vi "MTS_ToColorImage.vi"(0 "Data In":u32[](array[numeric]), 1 "Reset":bool, 2 "Image Array In":i32[][][](array[numeric]), 5 "Data Count":i32, 7 "TCSPC Binning":i32[][](array[numeric]), 9 "Pixel Time (Laser Pulses)":i32, 11 "Trace Bins":i32=25) -> (3 "Image Array Out":i32[][][](array[numeric]), 6 "Total Photon Count":u64[](array[numeric]), 8 "Trigger Times":u64[](array[numeric]), 13 "Total Oveflow Count":u64, 14 "Num Records Total":i32, 15 "Traces":i32[][](array[numeric]))   [LabVIEW 8.6]
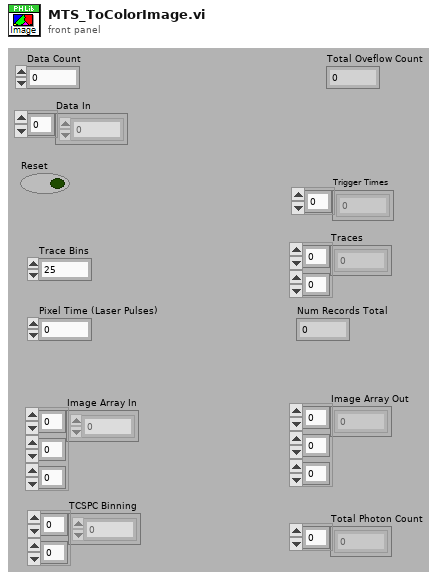
[diagram p1: front panel]
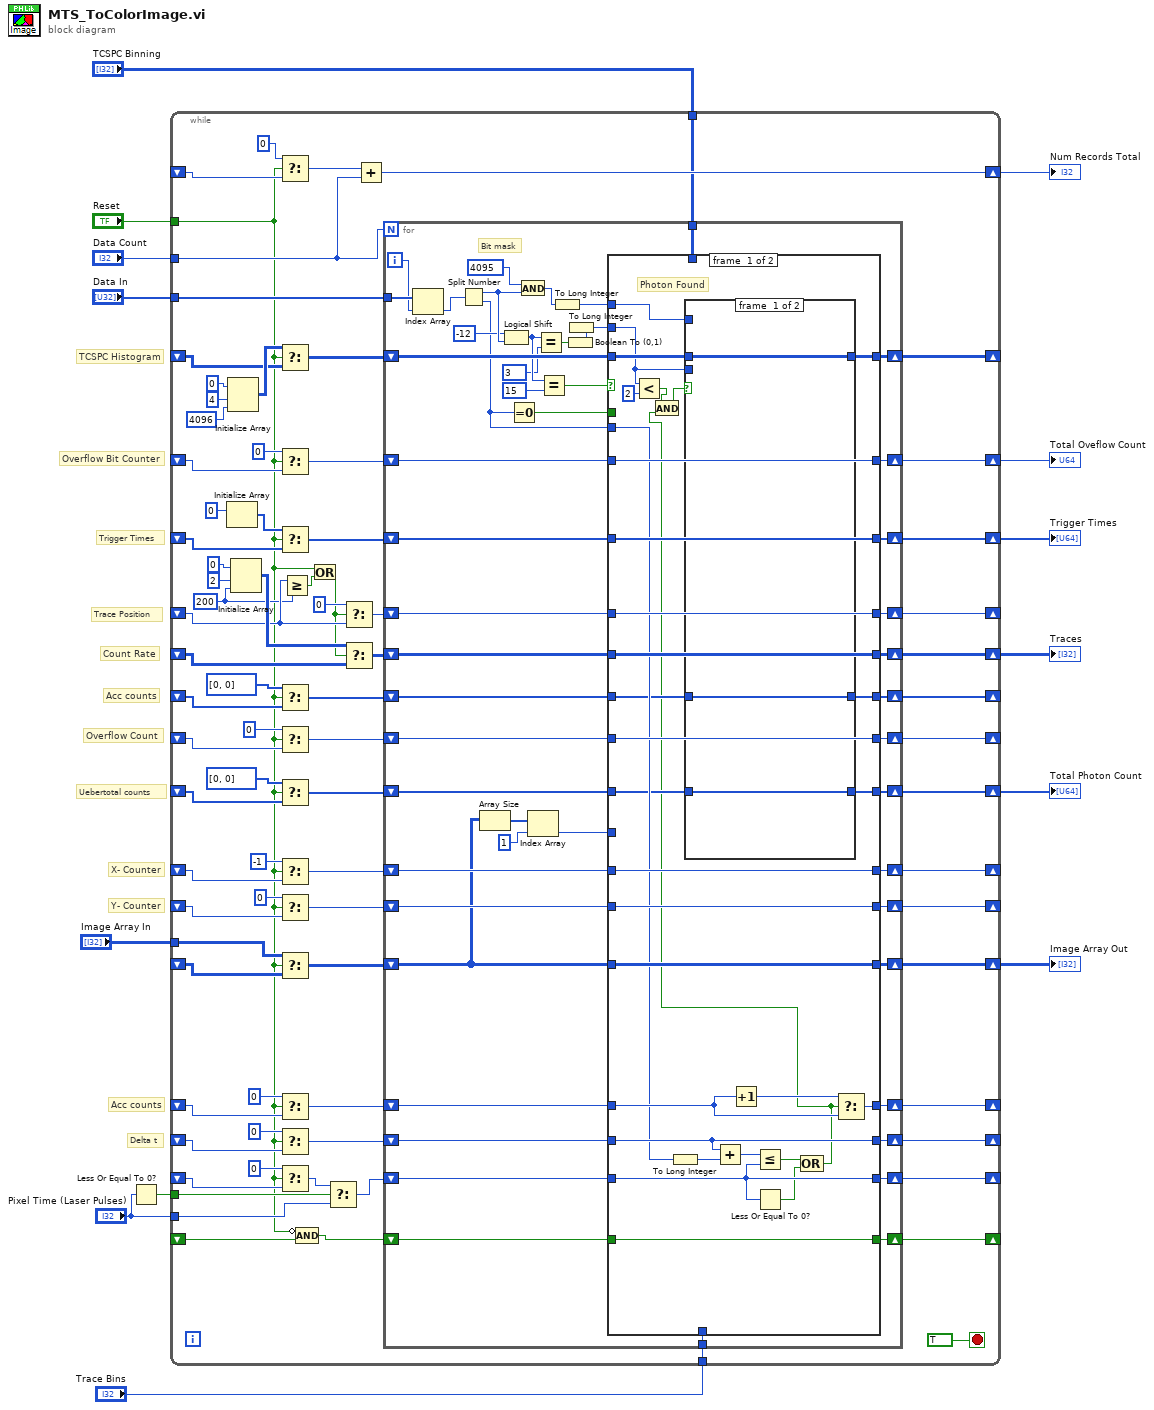
[diagram p0: block diagram]
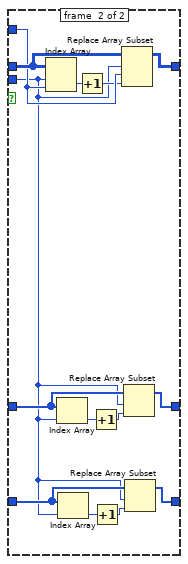
[diagram p2: hidden frame]
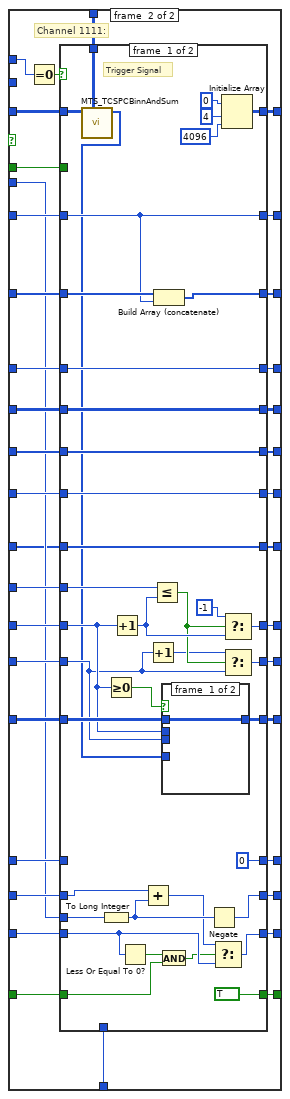
[diagram p3: hidden frame]
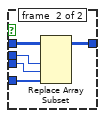
[diagram p4: hidden frame]
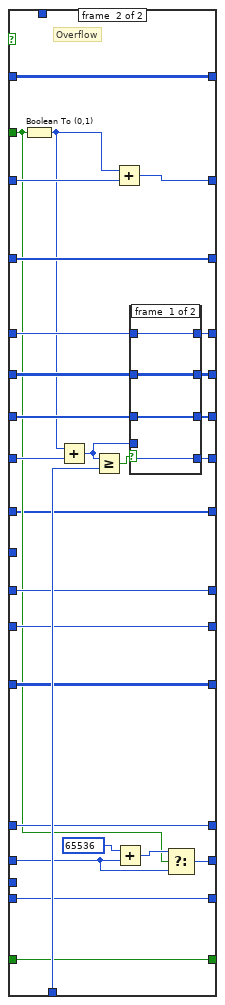
[diagram p5: hidden frame]
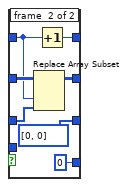
[diagram p6: hidden frame]
diagram:
  # "Uebertotal counts"
  # "Y- Counter"
  # "X- Counter"
  # "Delta t"
  # "Acc counts"
  # "Trace Position"
  # "Overflow Count"
  # "Acc counts"
  # "Count Rate"
  # "Trigger Times"
  # "TCSPC Histogram"
  # "Overflow Bit Counter"
  n1 = Less Or Equal To 0?(x="Pixel Time (Laser Pulses)") -> (x <= 0?=w3:bool)
  n2 = while {
    tunnel: "Data In" -> [w93]
    shift-right: [w94] -> _
    shift-left: _ -> [w89]
    tunnel: "Reset" -> [w16]
    shift-right: [w86] -> w5
    shift-left: _ -> [w85]
    shift-right: [w81] -> w12
    shift-left: _ -> [w80]
    shift-right: [w76] -> w10
    shift-left: _ -> [w75]
    shift-right: [w73] -> _
    shift-left: _ -> [w72]
    shift-right: [w70] -> _
    shift-left: _ -> [w69]
    tunnel: "Trace Bins" -> [w68]
    shift-right: [w65] -> _
    shift-left: _ -> [w63]
    shift-right: [w59] -> w8
    shift-left: _ -> [w58]
    tunnel: "Image Array In" -> [w61]
    shift-right: [w54] -> _
    shift-left: _ -> [w52]
    shift-right: [w53] -> _
    shift-left: _ -> [w51]
    shift-right: [w46] -> _
    shift-left: _ -> [w44]
    shift-right: [w45] -> _
    shift-left: _ -> [w43]
    tunnel: "Data Count" -> [w38]
    shift-right: [w37] -> w6
    shift-left: _ -> [w40]
    shift-right: [w28] -> w4
    shift-left: _ -> [w27]
    shift-right: [w23] -> _
    shift-left: _ -> [w20]
    tunnel: w3 -> [w25]
    tunnel: "Pixel Time (Laser Pulses)" -> [w24]
    shift-right: [w19] -> _
    shift-left: _ -> [w18]
    tunnel: "TCSPC Binning" -> [w15]
    stop <- TRUE stop-if-true
    w34 = 200 ("dimension size")
    n3 = Initialize Array(u64 0 ("element")) -> (w83:u64[])  [unwired: 1 out]
    n4 = Initialize Array(0 ("element"), 4 ("dimension size"), 4096 ("dimension size")) -> (w90:i32[][])
    n5 = Initialize Array(0 ("element"), 2 ("dimension size"), w34) -> (w78:i32[][])
    n6 = Select(t=0 ("Data Count 2"), s=w16, f=w40) -> (s? t:f=w39:i32)
    n7 = Select(t=w90, s=w16, f=w89) -> (s? t:f=w91:i32[][])
    n8 = Select(t=u64 0, s=w16, f=w85) -> (s? t:f=w87:u64)
    n9 = Select(t=w83, s=w16, f=w80) -> (s? t:f=w82:u64[])
    n10 = Select(t=u32[] [0, 0] ("initialized array"), s=w16, f=w72) -> (s? t:f=w74:u32[])
    n11 = Select(t=u32 0, s=w16, f=w69) -> (s? t:f=w71:u32)
    n12 = Select(t=u64[] [0, 0] ("initialized array"), s=w16, f=w27) -> (s? t:f=w29:u64[])
    n13 = Select(t=-1, s=w16, f=w44) -> (s? t:f=w48:i32)
    n14 = Select(t=0, s=w16, f=w43) -> (s? t:f=w47:i32)
    n15 = Select(t=w61, s=w16, f=w58) -> (s? t:f=w60:i32[][][])
    n16 = Select(t=0, s=w16, f=w52) -> (s? t:f=w56:i32)
    n17 = Select(t=0, s=w16, f=w51) -> (s? t:f=w55:i32)
    n18 = Select(t=0, s=w16, f=w20) -> (s? t:f=w22:i32)
    n19 = Greater Or Equal?(x=w63, y=w34) -> (x >= y?=w64:bool)
    n20 = Compound Arithmetic op=AND(invert w16, w18) -> (w17:bool)
    n21 = Or(x=w16, y=w64) -> (x .or. y?=w62:bool)
    n22 = Select(t=w22, s=w25, f=w24) -> (s? t:f=w26:i32)
    n23 = Select(t=0, s=w62, f=w63) -> (s? t:f=w66:i32)
    n24 = Select(t=w78, s=w62, f=w75) -> (s? t:f=w77:i32[][])
    n25 = Add(x=w39, y=w38) -> (x+y=w37:i32)
    n26 = for {
      N: w38 -> [_]
      tunnel: w93 -> [w110]
      shift-right: [w143] -> w94
      shift-left: w91 -> [w145]
      shift-right: [w137] -> w86
      shift-left: w87 -> [w138]
      shift-right: [w135] -> w81
      shift-left: w82 -> [w136]
      shift-right: [w130] -> w76
      shift-left: w77 -> [w131]
      shift-right: [w132] -> w73
      shift-left: w74 -> [w133]
      shift-right: [w128] -> w70
      shift-left: w71 -> [w129]
      tunnel: w68 -> [w127]
      shift-right: [w125] -> w65
      shift-left: w66 -> [w126]
      shift-right: [w124] -> w59
      shift-left: w60 -> [w116]
      shift-right: [w122] -> w54
      shift-left: w56 -> [w123]
      shift-right: [w120] -> w53
      shift-left: w55 -> [w121]
      shift-right: [w117] -> w46
      shift-left: w48 -> [w118]
      shift-right: [w113] -> w45
      shift-left: w47 -> [w119]
      shift-right: [w101] -> w28
      shift-left: w29 -> [w102]
      shift-right: [w100] -> w23
      shift-left: w26 -> [w112]
      shift-right: [w99] -> w19
      shift-left: w17 -> [w98]
      tunnel: w15 -> [w96]
      i -> [w109]
      # "Bit mask"
      n27 = Index Array(array=w110, index=w109) -> (element=w108:u32)
      n28 = Split Number(x=w108) -> (hi(x)=w142:u16, lo(x)=w111:u16)
      n29 = Array Size(array=w116) -> (size(s)=w115:i32[])
      n30 = Logical Shift(y=i8 -12, x=w142) -> (x << y=w107:u16)
      n31 = Equal To 0?(x=w111) -> (x = 0?=w134:bool)
      n32 = And(x=u16 4095, y=w142) -> (x .and. y?=w146:u16)
      n33 = Index Array(array=w115, index=1) -> (element=w114:i32)
      n34 = Equal?(x=w107, y=u16 3) -> (x = y?=w105:bool)
      n35 = Equal?(x=w107, y=u16 15) -> (x = y?=w139:bool)
      n36 = To Long Integer(number=w146) -> (32bit integer=w144:i32)
      n37 = Boolean To (0,1)(Boolean=w105) -> (0, 1=w104:i16)
      n38 = To Long Integer(number=w104) -> (32bit integer=w103:i32)
      n39 = case shown="True" w139 {
        tunnel: w145 -> [w178 w198]
        tunnel: w144 -> [w161 w211]
        tunnel: [w177 w197] -> w143
        tunnel: w103 -> [w158 _]
        tunnel: w138 -> [w176 w231]
        tunnel: [w176 w230] -> w137
        tunnel: w136 -> [w175 w229]
        tunnel: [w175 w228] -> w135
        tunnel: w134 -> [_ w227]
        tunnel: w133 -> [w160 w225]
        tunnel: [w159 w221] -> w132
        tunnel: w131 -> [w174 w224]
        tunnel: [w174 w220] -> w130
        tunnel: w129 -> [w173 w226]
        tunnel: [w173 w222] -> w128
        tunnel: w127 -> [_ w223]
        tunnel: w126 -> [w172 w219]
        tunnel: [w172 w218] -> w125
        tunnel: w116 -> [w171 w216]
        tunnel: [w171 w217] -> w124
        tunnel: w123 -> [w170 w212]
        tunnel: [w169 w213] -> w122
        tunnel: w121 -> [w168 w215]
        tunnel: [w168 w214] -> w120
        tunnel: w119 -> [w167 w210]
        tunnel: w118 -> [w166 w209]
        tunnel: [w166 w208] -> w117
        tunnel: w114 -> [_ w207]
        tunnel: [w167 w206] -> w113
        tunnel: w112 -> [w154 w202]
        tunnel: w111 -> [w163 w205]
        tunnel: w102 -> [w156 w204]
        tunnel: [w155 w203] -> w101
        tunnel: [w154 w201] -> w100
        tunnel: [w151 w200] -> w99
        tunnel: w98 -> [w151 w199]
        tunnel: w96 -> [_ w196]
        frame #0 {
          # "Photon Found"
          n40 = Less?(x=w158, y=2) -> (x < y?=w150:bool)
          n41 = To Long Integer(number=w163) -> (32bit integer=w162:i32)
          n42 = Add(x=w168, y=w162) -> (x+y=w164:i32)
          n43 = Increment(x=w170) -> (x+1=w165:i32)
          n44 = Less Or Equal?(x=w164, y=w154) -> (x <= y?=w153:bool)
          n45 = Less Or Equal To 0?(x=w154) -> (x <= 0?=w152:bool)
          n46 = Compound Arithmetic op=OR(w153, w152) -> (w148:bool)
          n47 = And(x=w150, y=w148) -> (x .and. y?=w149:bool)
          n48 = case shown="True" w149 {
            tunnel: w178 -> [w181 w195]
            tunnel: [w181 w194] -> w177
            tunnel: w161 -> [_ w193]
            tunnel: w158 -> [_ w182]
            tunnel: w160 -> [w180 w192]
            tunnel: [w180 w191] -> w159
            tunnel: w156 -> [w179 w184]
            tunnel: [w179 w183] -> w155
            frame #0 {
            }
            frame #1 {
              n49 = Index Array(array=w195, index (row)=w182, index (col)=w193) -> (element=w190:i32)
              n50 = Index Array(array=w192, index=w182) -> (element=w188:u32)
              n51 = Index Array(array=w184, index=w182) -> (element=w186:u64)
              n52 = Increment(x=w190) -> (x+1=w189:i32)
              n53 = Increment(x=w188) -> (x+1=w187:u32)
              n54 = Increment(x=w186) -> (x+1=w185:u64)
              n55 = Replace Array Subset(array=w195, new element=w189, index (row)=w182, index (col)=w193) -> (w194:i32[][])
              n56 = Replace Array Subset(array=w192, new element=w187, index=w182) -> (w191:u32[])
              n57 = Replace Array Subset(array=w184, new element=w185, index=w182) -> (w183:u64[])
            }
          }
          n58 = Select(t=w165, s=w148, f=w170) -> (s? t:f=w169:i32)
        }
        frame #1 {
          # "Channel 1111:"
          n59 = Equal To 0?(x=w211) -> (x = 0?=w232:bool)
          n60 = case shown="False" w232 {
            tunnel: w231 -> [w269 w304]
            tunnel: [w269 w303] -> w230
            tunnel: w229 -> [w271 w305]
            tunnel: [w270 w305] -> w228
            tunnel: w227 -> [_ w282]
            tunnel: w226 -> [w268 w288]
            tunnel: w225 -> [w267 w299]
            tunnel: w224 -> [w266 w297]
            tunnel: w223 -> [_ w302]
            tunnel: [w268 w300] -> w222
            tunnel: [w267 w298] -> w221
            tunnel: [w266 w296] -> w220
            tunnel: w219 -> [w265 w295]
            tunnel: [w265 w294] -> w218
            tunnel: [w263 w293] -> w217
            tunnel: w216 -> [w264 w293]
            tunnel: w215 -> [w249 w283]
            tunnel: [w251 w284] -> w214
            tunnel: [0 ("t") w291] -> w213
            tunnel: w212 -> [_ w291]
            tunnel: w205 -> [w248 _]
            tunnel: w210 -> [w253 w290]
            tunnel: w209 -> [w258 w289]
            tunnel: [w260 w289] -> w208
            tunnel: w207 -> [w259 _]
            tunnel: [w254 w290] -> w206
            tunnel: w204 -> [w250 w281]
            tunnel: [w250 w281] -> w203
            tunnel: w202 -> [w245 w280]
            tunnel: [w244 w280] -> w201
            tunnel: [TRUE w279] -> w200
            tunnel: w199 -> [w240 w279]
            tunnel: w198 -> [w235 w278]
            tunnel: [w236 w278] -> w197
            tunnel: w196 -> [w234 _]
            frame #0 {
              # "Trigger Signal"
              n61 = call "MTS_TCSPCBinnAndSum.vi"("TCSPC Binning"=w234, "TCSPC Histogram"=w235) -> ("Intensity Values"=w233:i32[])  [unwired: 1 in, 8 out]
              n62 = To Long Integer(number=w248) -> (32bit integer=w247:i32)
              n63 = Greater Or Equal To 0?(x=w258) -> (x >= 0?=w261:bool)
              n64 = Increment(x=w258) -> (x+1=w257:i32)
              n65 = Less Or Equal To 0?(x=w245) -> (x <= 0?=w243:bool)
              n66 = Add(x=w249, y=w247) -> (x+y=w246:i32)
              n67 = Increment(x=w253) -> (x+1=w252:i32)
              n68 = Less Or Equal?(x=w259, y=w257) -> (x <= y?=w255:bool)
              n69 = Build Array (concatenate)(w271, w269) -> (w270:u64[])
              n70 = And(x=w243, y=w240) -> (x .and. y?=w242:bool)
              n71 = case shown="True" w261 {
                tunnel: w264 -> [w272 w277]
                tunnel: [w272 w276] -> w263
                tunnel: w253 -> [_ w275]
                tunnel: w258 -> [_ w274]
                tunnel: w233 -> [_ w273]
                frame #0 {
                }
                frame #1 {
                  n72 = Replace Array Subset(array=w277, new element=w273, index (dim 1)=w274, index (dim 2)=w275) -> (w276:i32[][][])  [unwired: 1 in]
                }
              }
              n73 = Negate(x=w247) -> (-x=w251:i32)
              n74 = Select(t=w246, s=w242, f=w245) -> (s? t:f=w244:i32)
              n75 = Initialize Array(0 ("element"), 4 ("dimension size"), 4096 ("dimension size")) -> (w236:i32[][])
              n76 = Select(t=-1, s=w255, f=w257) -> (s? t:f=w260:i32)
              n77 = Select(t=w252, s=w255, f=w253) -> (s? t:f=w254:i32)
            }
            frame #1 {
              # "Overflow"
              n78 = Boolean To (0,1)(Boolean=w282) -> (0, 1=w286:i16)
              n79 = Add(x=w286, y=w288) -> (x+y=w287:u32)
              n80 = Greater Or Equal?(x=w287, y=w302) -> (x >= y?=w301:bool)
              n81 = Add(x=w286, y=w304) -> (x+y=w303:u64)
              n82 = Add(x=65536 ("t"), y=w283) -> (x+y=w285:i32)
              n83 = case shown="True" w301 {
                tunnel: w287 -> [w309 _]
                tunnel: [w309 u32 0] -> w300
                tunnel: w299 -> [w308 w314]
                tunnel: [w308 u32[] [0, 0] ("initialized array")] -> w298
                tunnel: w297 -> [w307 w315]
                tunnel: [w307 w313] -> w296
                tunnel: w295 -> [w306 w311]
                tunnel: [w306 w312] -> w294
                frame #0 {
                }
                frame #1 {
                  n84 = Replace Array Subset(array=w315, new element=w314, index (col)=w311) -> (w313:i32[][])  [unwired: 1 in]
                  n85 = Increment(x=w311) -> (x+1=w312:i32)
                }
              }
              n86 = Select(t=w285, s=w282, f=w283) -> (s? t:f=w284:i32)
            }
          }
        }
      }
    }
  }
  "Trigger Times" <- w12
  "Traces" <- w10
  "Image Array Out" <- w8
  "Num Records Total" <- w6
  "Total Oveflow Count" <- w5
  "Total Photon Count" <- w4
